vi "Calculate Sweep Values.vi"(7 "Sweep type":string, 8 "error in":errorcluster, 9 "Points":i32, 10 "Stop level":dbl, 11 "Start level":dbl) -> (0 "error out":errorcluster, 2 "Sweep points":i32, 3 "Sweep values":dbl[](array[numeric]))   [LabVIEW 2024]
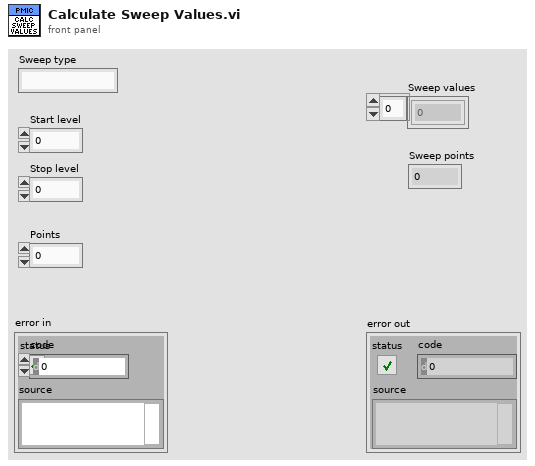
[diagram p1: front panel]
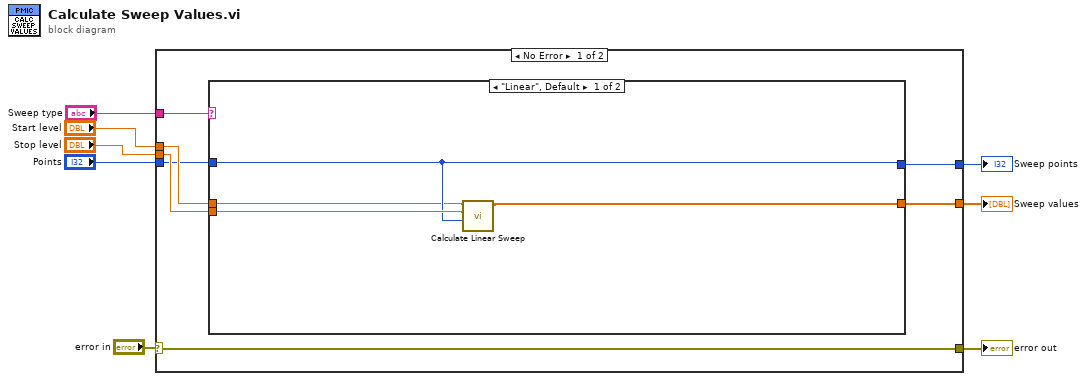
[diagram p0: block diagram]
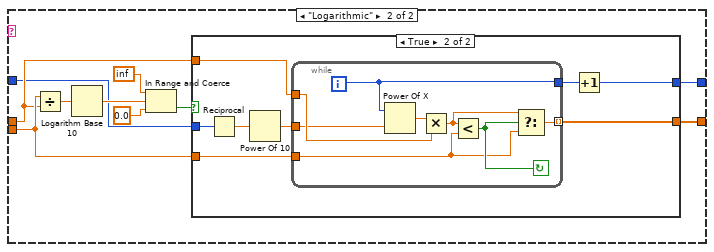
[diagram p2: hidden frame]
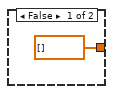
[diagram p3: hidden frame]
diagram:
  n1 = case shown="No Error" "error in" {
    selector: "error in" -> [w10 w47]
    tunnel: [w12 _] -> w7
    tunnel: "Points" -> [w13 _]
    tunnel: "Start level" -> [w15 _]
    tunnel: "Stop level" -> [w14 _]
    tunnel: [w10 w47] -> w3
    tunnel: "Sweep type" -> [w11 _]
    tunnel: [w9 _] -> w1
    frame No Error {
      n2 = case shown="\"Linear\", Default" w11 {
        tunnel: w13 -> [w18 w20]
        tunnel: [w16 w24] -> w12
        tunnel: w15 -> [w17 w21]
        tunnel: w14 -> [w19 w28]
        tunnel: [w18 w25] -> w9
        frame "Linear", Default {
          n3 = call "Calculate Linear Sweep.vi"("Points"=w18, "Stop level"=w19, "Start level"=w17) -> ("Values"=w16:dbl[])  [unwired: 8 in]
        }
        frame "Logarithmic" {
          n4 = Divide(x=w28, y=w21) -> (x/y=w29:dbl)
          n5 = Logarithm Base 10(1:w29) -> (0:w26:dbl)
          n6 = In Range and Coerce(upper limit=inf, x=w26, lower limit=0.0) -> (In Range?=w23:bool)  [unwired: 1 out]
          n7 = case shown="True" w23 {
            tunnel: [dbl[] [] w38] -> w24
            tunnel: [_ w31] -> w25
            tunnel: w28 -> [_ w37]
            tunnel: w21 -> [_ w36]
            tunnel: w20 -> [_ w33]
            frame False {
            }
            frame True {
              n8 = Reciprocal(x=w33) -> (1/x=w35:dbl)
              n9 = Power Of 10(x=w35) -> (10^x=w34:dbl)
              n10 = while {
                tunnel: w34 -> [w43]
                tunnel: w36 -> [w46]
                tunnel: [w42] -> w38 mode=indexing
                tunnel: [w44] -> w32
                tunnel: w37 -> [w39]
                i -> [w44]
                stop <- w41 continue-if-true
                n11 = Power Of X(1:w43, 2:w44) -> (0:w45:dbl)
                n12 = Multiply(x=w45, y=w46) -> (x*y=w40:dbl)
                n13 = Less?(x=w40, y=w39) -> (x < y?=w41:bool)
                n14 = Select(t=w40, s=w41, f=w39) -> (s? t:f=w42:dbl)
              }
              n15 = Increment(x=w32) -> (x+1=w31:i32)
            }
          }
        }
      }
    }
    frame Error {
    }
  }
  "Sweep values" <- w7
  "error out" <- w3
  "Sweep points" <- w1
